vi "XBOX and Joystick Control.vi"(1 "Left Joystick":cluster{"Axes":dbl[], "Buttons":bool[]}, 2 "XBOX":T1, 3 "Right Joystick":cluster{"Axes":dbl[], "Buttons":bool[]}) -> ()   [LabVIEW 2018]
uses:
  <vilib>/Rock Robotics/WPI/ThirdParty/Sensors/navX/_TypeDefs/FRIC_navX_DeviceNumbersTypeDef.ctl
  Robot Global Data.vi
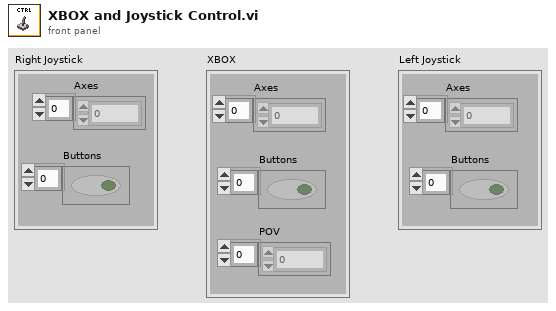
[diagram p1: front panel]
types:
  T1 = cluster{"Axes":dbl[], "Buttons":bool[], "POV":i16[]}
  T2 = typedef "FRIC_navX_DeviceNumbersTypeDef.ctl" = enum16{"Dev0", "Dev1", "Dev2", "Dev3"}
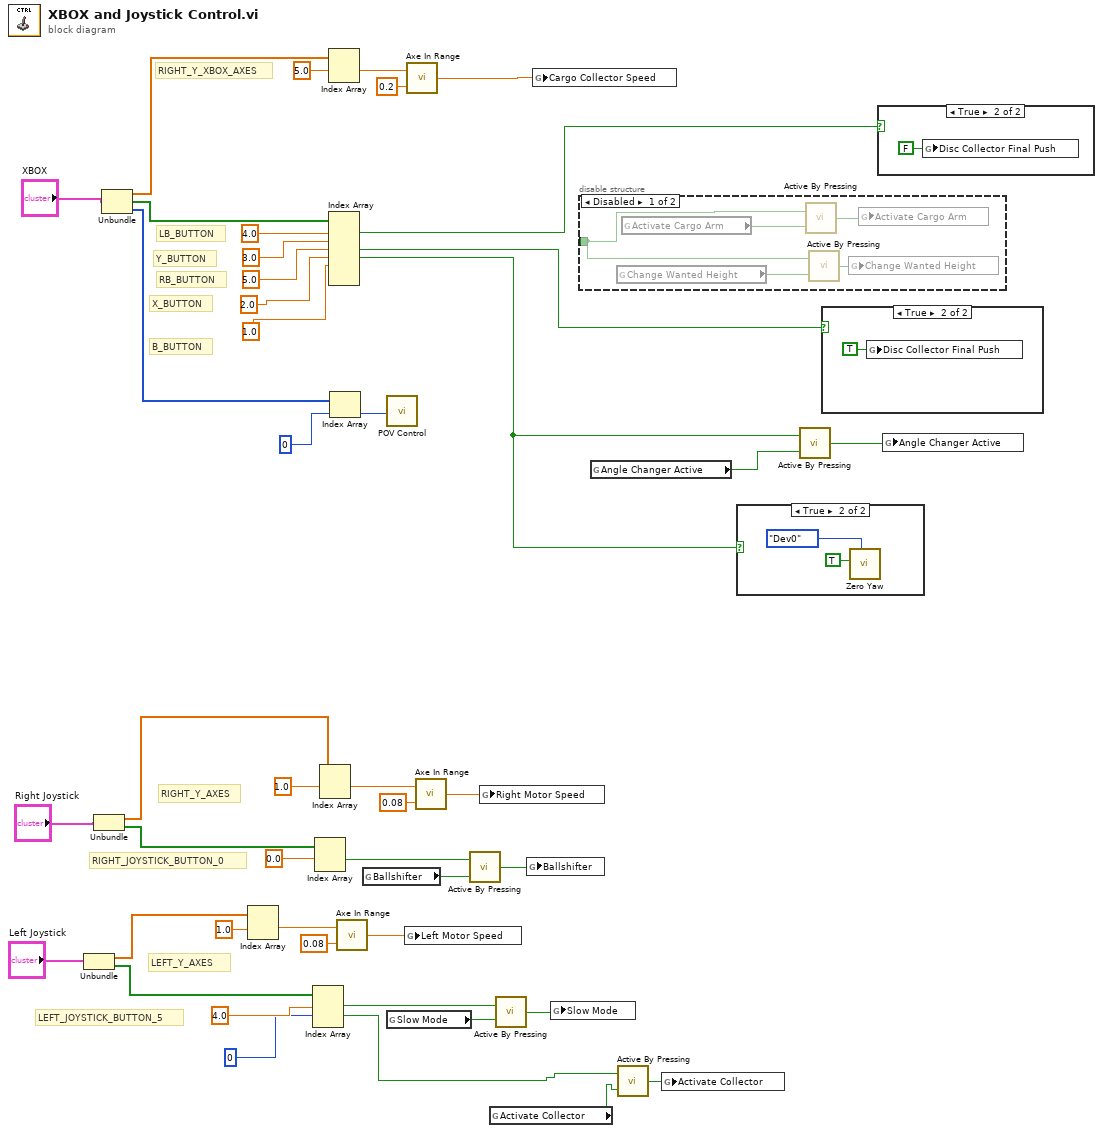
[diagram p0: block diagram]
diagram:
  # "B_BUTTON"
  # "LEFT_JOYSTICK_BUTTON_5"
  # "LEFT_Y_AXES"
  # "RIGHT_JOYSTICK_BUTTON_0"
  # "RIGHT_Y_AXES"
  # "X_BUTTON"
  # "RB_BUTTON"
  # "RIGHT_Y_XBOX_AXES"
  # "Y_BUTTON"
  # "LB_BUTTON"
  n1 = Unbundle("Left Joystick") -> ("Axes"=w32:dbl[], "Buttons"=w31:bool[])
  n2 = Unbundle("Right Joystick") -> ("Axes"=w34:dbl[], "Buttons"=w33:bool[])
  n3 = Unbundle("XBOX") -> ("Axes"=w45:dbl[], "Buttons"=w44:bool[], "POV"=w13:i16[])
  n4 = Index Array(array=w32, index #1=1.0) -> (element #1=w18:dbl)  [unwired: 1 in, 1 out]
  n5 = Index Array(array=w31, index #1=4.0, index #2=0 ("index")) -> (element #1=w26:bool, element #2=w3:bool)  [unwired: 1 in, 1 out]
  n6 = Index Array(array=w33, index #1=0.0) -> (element #1=w30:bool)  [unwired: 1 in, 1 out]
  n7 = Index Array(array=w34, index #1=1.0) -> (element #1=w19:dbl)  [unwired: 1 in, 1 out]
  n8 = Index Array(array=w45, index #1=5.0) -> (element #1=w43:dbl)  [unwired: 1 in, 1 out]
  n9 = Index Array(array=w44, index #1=4.0 ("Y_BUTTON"), index #2=3.0, index #3=5.0, index #4=2.0, index #5=1.0) -> (element #1=w9:bool, element #3=w10:bool, element #4=w7:bool)  [unwired: 2 in, 4 out]
  n10 = Index Array(array=w13, index=0) -> (element=w11:i16)
  n11 = call "Axe In Range.vi"("RangeNumber"=0.08, "Axe"=w18) -> ("NumericGlobalData"=w17:dbl)
  n12 = global read "Robot Global Data.vi" "Ballshifter"() -> (w29:bool)
  n13 = call "POV Control.vi"("POV Number"=w11) -> ()  [unwired: 1 in]
  n14 = global read "Robot Global Data.vi" "Slow Mode"() -> (w27:bool)
  n15 = global write "Robot Global Data.vi" "Left Motor Speed"(w17) -> ()
  n16 = call "Axe In Range.vi"("RangeNumber"=0.2, "Axe"=w43) -> ("NumericGlobalData"=w8:dbl)
  n17 = call "Axe In Range.vi"("RangeNumber"=0.08, "Axe"=w19) -> ("NumericGlobalData"=w15:dbl)
  n18 = call "Active By Pressing.vi"("Global Data Name 1"=w29, "Button Press"=w30) -> ("Global Data Name 2"=w25:bool)
  n19 = global write "Robot Global Data.vi" "Right Motor Speed"(w15) -> ()
  n20 = global read "Robot Global Data.vi" "Activate Collector"() -> (w1:bool)
  n21 = call "Active By Pressing.vi"("Global Data Name 1"=w27, "Button Press"=w26) -> ("Global Data Name 2"=w28:bool)
  n22 = global write "Robot Global Data.vi" "Ballshifter"(w25) -> ()
  n23 = global write "Robot Global Data.vi" "Cargo Collector Speed"(w8) -> ()
  n24 = global write "Robot Global Data.vi" "Slow Mode"(w28) -> ()
  n25 = disable-structure shown="Disabled" {
    disable-tunnel: _ -> [w47 _]
    frame Disabled {
      n26 = global read "Robot Global Data.vi" "Change Wanted Height"() -> (w48:bool)
      n27 = global read "Robot Global Data.vi" "Activate Cargo Arm"() -> (w50:bool)
      n28 = call "Active By Pressing.vi"("Global Data Name 1"=w50, "Button Press"=w47) -> ("Global Data Name 2"=w51:bool)
      n29 = call "Active By Pressing.vi"("Global Data Name 1"=w48, "Button Press"=w47) -> ("Global Data Name 2"=w49:bool)
      n30 = global write "Robot Global Data.vi" "Change Wanted Height"(w49) -> ()
      n31 = global write "Robot Global Data.vi" "Activate Cargo Arm"(w51) -> ()
    }
    frame Enabled {
    }
  }
  n32 = global read "Robot Global Data.vi" "Angle Changer Active"() -> (w20:bool)
  n33 = call "Active By Pressing.vi"("Global Data Name 1"=w1, "Button Press"=w3) -> ("Global Data Name 2"=w2:bool)
  n34 = global write "Robot Global Data.vi" "Activate Collector"(w2) -> ()
  n35 = case shown="True" w7 {
    frame False {
    }
    frame True {
      n36 = call <vilib>:"Zero Yaw.vi"("Device Number"=FRIC_navX_DeviceNumbersTypeDef."Dev0", "Zero"=TRUE) -> ()  [unwired: 10 in]
    }
  }
  n37 = call "Active By Pressing.vi"("Global Data Name 1"=w20, "Button Press"=w7) -> ("Global Data Name 2"=w37:bool)
  n38 = case shown="True" w10 {
    frame False {
    }
    frame True {
      n39 = global write "Robot Global Data.vi" "Disc Collector Final Push"(TRUE ("Disc Collector Final Push")) -> ()
    }
  }
  n40 = case shown="True" w9 {
    frame False {
    }
    frame True {
      n41 = global write "Robot Global Data.vi" "Disc Collector Final Push"(FALSE ("Disc Collector Final Push")) -> ()
    }
  }
  n42 = global write "Robot Global Data.vi" "Angle Changer Active"(w37) -> ()
